vi "ColumbiaSonicareOld.vi"() -> ()   [LabVIEW 2022 SP3]
uses:
  Doppler data processing/Doppler/dopplerV6.llb/AI Waveform Scan (waveform).vi
  Doppler data processing/Doppler/dopplerV6.llb/AI Read (waveform).vi
  <vilib>/sound/lvsound.llb/Sound Format.ctl
panel:
  in  "Case Constant\n(See Context Help)":bool=TRUE
  in  "Mode":enum32{"HIFU", "Thromb"}(tab)
  out "Exp Count":i32
  in  "Time between exposures (s)":sgl=2.2 min=0 format="%.1f"
  in  "Number of Exposures":i32=1 min=1
  in  "Therapy Duration (s)":dbl=0.1 min=0.1 max=10.0 step=0.1 format="%.1f"
  out "Time":i32=1 min=1
  out "PRF time  (ms)":sgl format="%.3f"
  in  "exp per cycle  (ms)":sgl=0.5 format="%.3f"
  in  "Total  Time On (s)":sgl=1.0 min=0.001 format="%.2f"
  out "PRF  (kHz)":sgl=1.0 min=0.001 format="%.3f"
  in  "Duty Cycle":sgl=0.5 min=0 max=1 format="%.2f"
  in  "EKG ?":bool=TRUE
  in  "Re-Zero Trig":bool
  out "waveform data":waveform(dbl)[](array[waveform])
  in  "New EKG (F1)":bool
  in  "Exit Program (F2)":bool
  out "EKG":waveform(dbl)[](graph)
  in  "Fire Therapy (ESC)":bool
  out "Therapy Delay (s)":dbl=1.0 format="%.3f"
  # "1. Select EKG mode with switch below.\n2. If in EKG mode, update EKG trace with New EKG (F1).\n3. Drag pink line to mark start time of exposure and trigger level.\n4. Set time duration of exposure (0.1 s steps).\n5. Choose number of exposures and time between exposures (2.2 s min in EKG mode)..\n6. Start exposure with Fire Therapy (ESC) (Green means on).\n7. Press Fire Therapy (ESC) again for emergency stop (Red means off).\n8. To exit program, Press Exit Program (F2) to  terminate program.\n9. Thromb tab permits exposures of a fixed PRF, duty cycle, and time duration. EKG  is\n     inactive when Thromb is selected."
  # "© 2003 Riverside Research Institute"
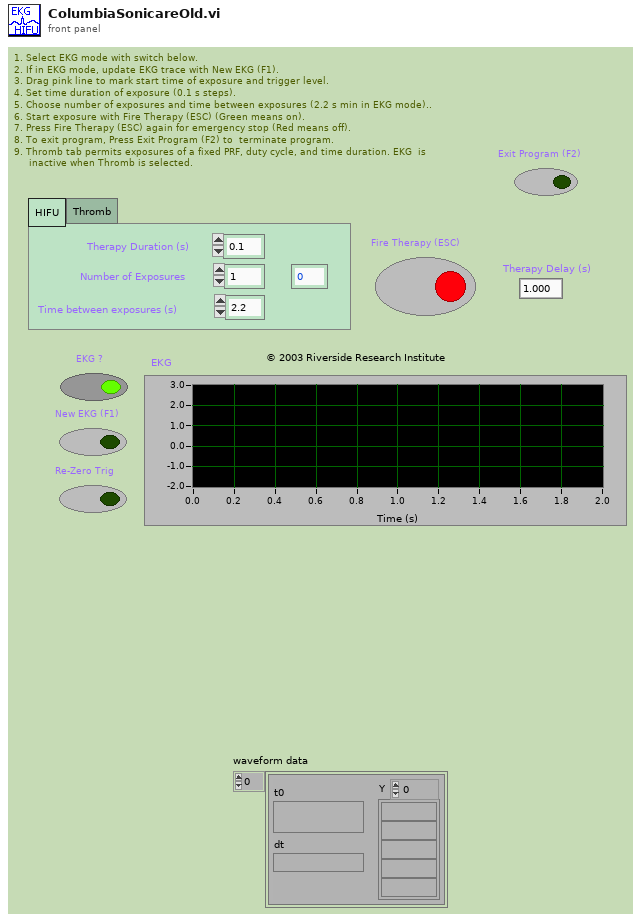
[diagram p1: front panel]
types:
  T1 = enum16{"setup mode 0", "setup mode 1", "setup mode 2", "setup mode 3", "setup mode 4", "setup mode 5", "read", "reset"}
  T2 = cluster{"coupling (no change:0)":enum16{"no change", "DC", "AC", "GND", "internal ref."}, "input config (no change:0)":u16}[]
  T3 = cluster{"high limit (0.0)":sgl, "low limit (0.0)":sgl}[]
  T4 = cluster{"trigger type (no trig:0)":enum16{"no trigger", "analog", "digital A", "digital B", "scan clock gate", "software analog "}, "pretrigger scans (0)":i32, "edge or slope \n(no change)":enum16{"no change", "rising", "falling"}, "analog chan (-) & level (0.0)":cluster{"trigger channel (empty)":string, "level (0.0)":sgl}, "scan clock source\n(no change:0)":enum16{"no change", "internal", "I/O Connector", "RTSI"}}
  T5 = typedef "Sound Format.ctl" = cluster{"sound quality":enum16{"mono", "stereo"}, "rate":enum16{"11025", "22050", "44100", "8000"}, "bits per sample":enum16{"8 bit", "16 bit"}}
  T6 = enum16{"ungated/software start", "count while high", "count while low", "start on rising edge", "start on falling edge"}
  T7 = enum16{"no trigger", "analog", "digital A", "digital A & B", "scan clock gate"}
  T8 = cluster{"trigger channel (empty)":string, "Cursor.Cursor Y":dbl}
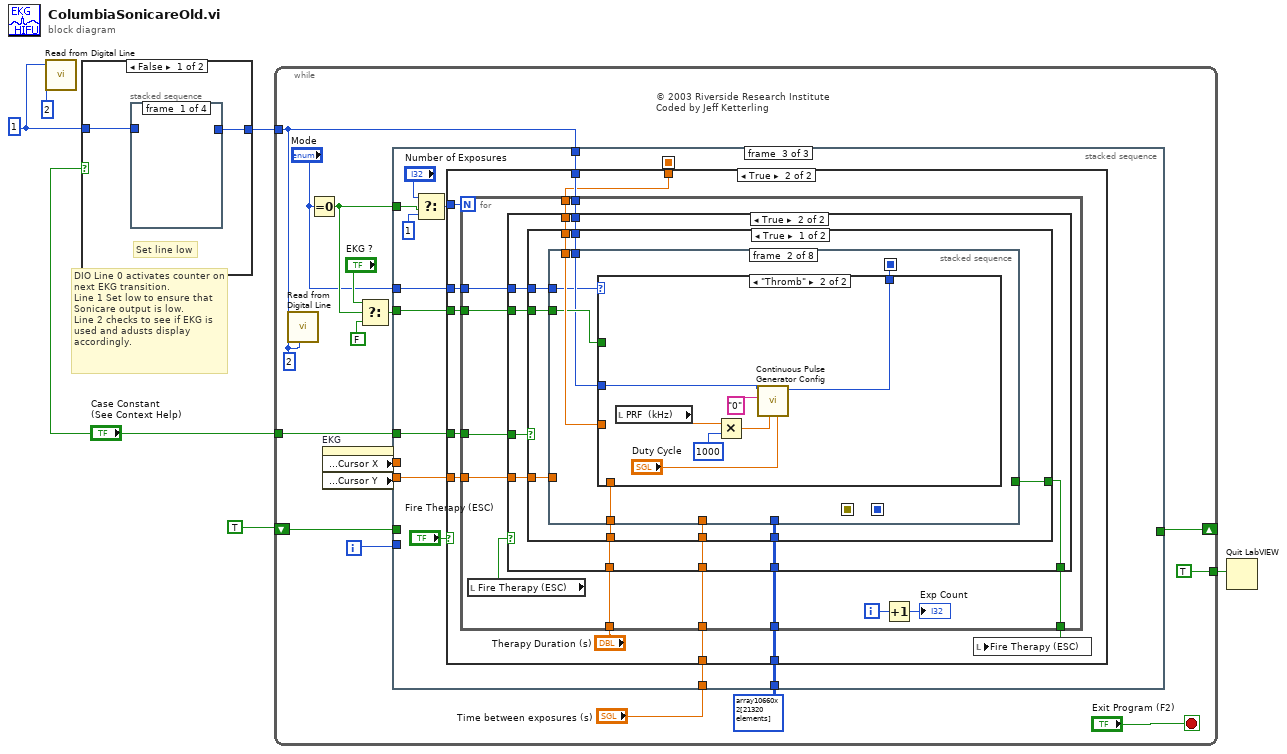
[diagram p0: block diagram]
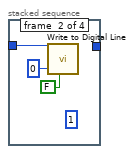
[diagram p2: hidden frame]
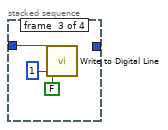
[diagram p3: hidden frame]
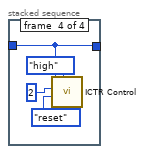
[diagram p4: hidden frame]
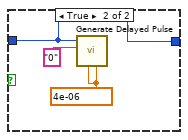
[diagram p5: hidden frame]
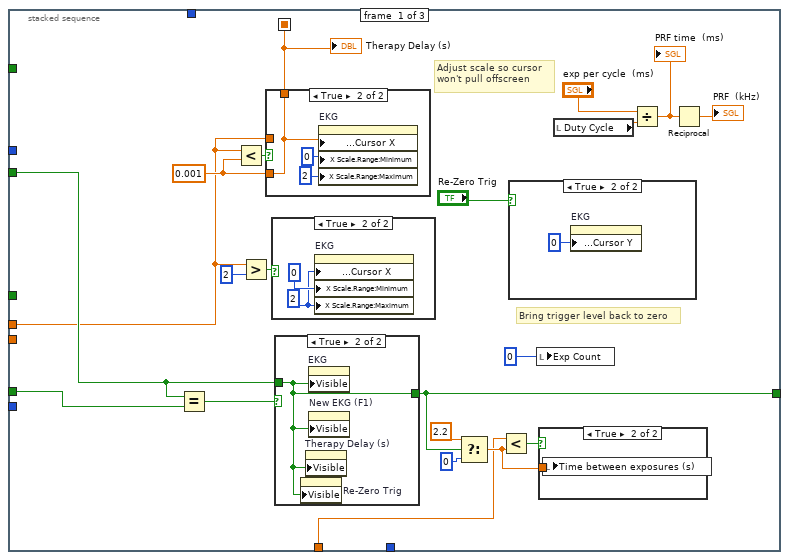
[diagram p6: hidden frame]
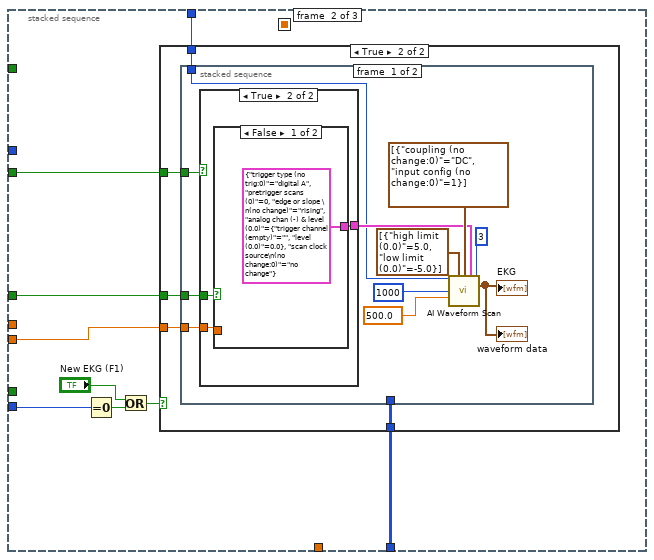
[diagram p12: hidden frame]
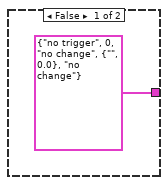
[diagram p14: hidden frame]
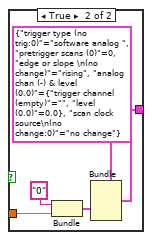
[diagram p15: hidden frame]
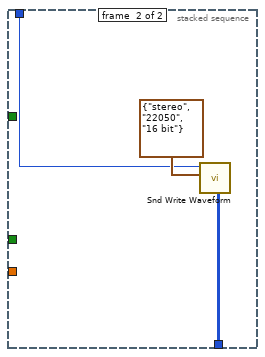
[diagram p16: hidden frame]
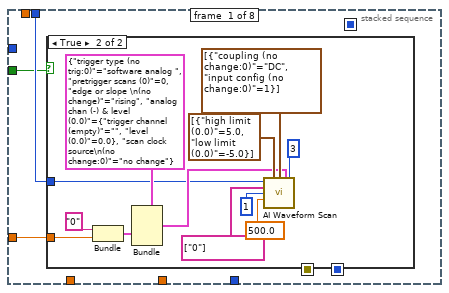
[diagram p19: hidden frame]
diagram:
  w1 = 1
  # "DIO Line 0 activates counter on next EKG transition.\nLine 1 Set low to ensure that Sonicare output is low.\nLine 2 checks to see if EKG is used and adusts display accordingly."
  n1 = call <vilib>:"Read from Digital Line.vi"("device"=w1, "line"=2) -> ()  [unwired: 5 in, 1 out]
  n2 = case shown="False" "Case Constant\n(See Context Help)" {
    tunnel: [w8 w21] -> w5
    tunnel: w1 -> [w7 w21]
    frame False {
      # "Set line low"
      n3 = stacked-sequence {
        tunnel: [_ _ _ w15] -> w8
        tunnel: w7 -> [_ w9 w13 w15]
        frame #0 {
        }
        frame #1 {
          (unwired) 1
          n4 = call <vilib>:"Write to Digital Line.vi"("device"=w9, "line"=0, "line state"=FALSE) -> ()  [unwired: 6 in]
        }
        frame #2 {
          n5 = call <vilib>:"Write to Digital Line.vi"("device"=w13, "line"=1, "line state"=FALSE) -> ()  [unwired: 6 in]
        }
        frame #3 {
          n6 = call <vilib>:"ICTR Control.vi"("output state"=enum16{"low", "high"}."high", "control code"=T1."reset", "counter"=i16 2, "device"=w15) -> ()  [unwired: 6 in, 2 out]
        }
      }
    }
    frame True {
      w19 = 4e-06
      n7 = call <vilib>:"Generate Delayed Pulse.vi"("pulse width (s or cycles)"=w19, "pulse delay (s or cycles)"=w19, "counter"="0", "device"=w21) -> ()  [unwired: 5 in, 3 out]
    }
  }
  n8 = while {
    tunnel: w5 -> [w34]
    shift-right: [w35] -> _
    shift-left: TRUE -> [w36]
    tunnel: [TRUE] -> w4
    tunnel: "Case Constant\n(See Context Help)" -> [w31]
    i -> [w37]
    stop <- "Exit Program (F2)" stop-if-true
    w32 = 2
    # "© 2003 Riverside Research Institute\nCoded by Jeff Ketterling"
    n9 = call <vilib>:"Read from Digital Line.vi"("device"=w34, "line"=w32, "iteration (0:initialize)"=w32) -> ()  [unwired: 4 in, 1 out]
    n10 = Equal To 0?(x="Mode") -> (x = 0?=w23:bool)
    n11 = property on="EKG" class="WFGraph (strict)"() -> ("Cursor.Cursor Position:Cursor X"=w29:dbl, "Cursor.Cursor Position:Cursor Y"=w30:dbl)  [unwired: 2 in, 2 out]
    n12 = Select(t="EKG ?", s=w23, f=FALSE) -> (s? t:f=w25:bool)
    n13 = stacked-sequence {
      seq-local: [w58 _ _] -> [_ _ w118]
      tunnel: w34 -> [_ w78 w120]
      tunnel: w37 -> [_ w77 _]
      tunnel: w25 -> [w54 w73 w119]
      tunnel: w36 -> [w53 _ _]
      tunnel: [w45 _ _] -> w35
      tunnel: w31 -> [_ w72 w117]
      tunnel: w30 -> [_ w71 w116]
      tunnel: w29 -> [w51 _ _]
      tunnel: i16[][] array10660x2[21320 elements] ("stereo 16-bit") -> [_ w70 w115]
      tunnel: "Time between exposures (s)" -> [w44 _ w114]
      tunnel: w23 -> [_ _ w111]
      tunnel: "Mode" -> [_ _ w108]
      frame #0 {
        w57 = 0.001
        # "Bring trigger level back to zero"
        # "Adjust scale so cursor won't pull offscreen"
        n14 = Equal?(x=w54, y=w53) -> (x = y?=w52:bool)
        n15 = Less?(x=w51, y=w57) -> (x < y?=w59:bool)
        n16 = Greater?(x=w51, y=2) -> (0:w55:bool)
        n17 = case shown="True" w59 {
          tunnel: w51 -> [w66 _]
          tunnel: [w66 w69] -> w58
          tunnel: w57 -> [_ w69]
          frame False {
          }
          frame True {
            n18 = property on="EKG" class="WFGraph (strict)"("Cursor.Cursor Position:Cursor X"=w69, "X Scale.Range:Minimum"=0, "X Scale.Range:Maximum"=2) -> ()  [unwired: 2 in, 2 out]
          }
        }
        "Therapy Delay (s)" <- w58
        n19 = case shown="True" w55 {
          frame False {
          }
          frame True {
            w64 = 2
            n20 = property on="EKG" class="WFGraph (strict)"("Cursor.Cursor Position:Cursor X"=w64, "X Scale.Range:Minimum"=0, "X Scale.Range:Maximum"=w64) -> ()  [unwired: 2 in, 2 out]
          }
        }
        n21 = case shown="True" w52 {
          tunnel: w54 -> [w62 w63]
          tunnel: [w62 w63] -> w45
          frame False {
          }
          frame True {
            n22 = property on="Re-Zero Trig" class="Bool"("Visible"=w63) -> ()  [unwired: 2 in, 2 out]
            n23 = property on="Therapy Delay (s)" class="DigNum (strict)"("Visible"=w63) -> ()  [unwired: 2 in, 2 out]
            n24 = property on="EKG" class="WFGraph (strict)"("Visible"=w63) -> ()  [unwired: 2 in, 2 out]
            n25 = property on="New EKG (F1)" class="Bool"("Visible"=w63) -> ()  [unwired: 2 in, 2 out]
          }
        }
        n26 = Select(t=2.2, s=w45, f=0) -> (s? t:f=w46:dbl)
        n27 = Less?(x=w44, y=w46) -> (x < y?=w47:bool)
        n28 = case shown="True" "Re-Zero Trig" {
          frame False {
          }
          frame True {
            n29 = property on="EKG" class="WFGraph (strict)"("Cursor.Cursor Position:Cursor Y"=0) -> ()  [unwired: 2 in, 2 out]
          }
        }
        n30 = local write "Exp Count"(0) -> ()
        n31 = case shown="True" w47 {
          tunnel: w46 -> [_ w60]
          frame False {
          }
          frame True {
            n32 = local write "Time between exposures (s)"(w60) -> ()
          }
        }
        n33 = local read "Duty Cycle"() -> (w42:sgl)
        n34 = Divide(x="exp per cycle  (ms)", y=w42) -> (x/y=w40:sgl)
        "PRF time  (ms)" <- w40
        n35 = Reciprocal(x=w40) -> (1/x=→"PRF  (kHz)":sgl)
      }
      frame #1 {
        n36 = Equal To 0?(x=w77) -> (x = 0?=w76:bool)
        n37 = Or(x="New EKG (F1)", y=w76) -> (x .or. y?=w74:bool)
        n38 = case shown="True" w74 {
          tunnel: w78 -> [_ w82]
          tunnel: w73 -> [_ w83]
          tunnel: w72 -> [_ w81]
          tunnel: w71 -> [_ w80]
          tunnel: w70 -> [_ w79]
          frame False {
          }
          frame True {
            n39 = stacked-sequence {
              tunnel: w83 -> [w87 _]
              tunnel: w82 -> [w86 w105]
              tunnel: w81 -> [w85 _]
              tunnel: w80 -> [w84 _]
              tunnel: w79 -> [_ w106]
              frame #0 {
                n40 = case shown="True" w87 {
                  tunnel: [T4 {"trigger type (no trig:0)"=enum."no trigger", "pretrigger scans (0)"=0, "edge or slope \n(no change)"=enum."no change", "analog chan (-) & level (0.0)"={"trigger channel (empty)"="", "level (0.0)"=0.0}, "scan clock source\n(no change:0)"=enum."no change"} ("trigger and clock (no trig, int clk)") w98] -> w89
                  tunnel: w85 -> [_ w97]
                  tunnel: w84 -> [_ w96]
                  frame False {
                  }
                  frame True {
                    n41 = case shown="False" w97 {
                      tunnel: [T4 {"trigger type (no trig:0)"=enum."digital A", "pretrigger scans (0)"=0, "edge or slope \n(no change)"=enum."rising", "analog chan (-) & level (0.0)"={"trigger channel (empty)"="", "level (0.0)"=0.0}, "scan clock source\n(no change:0)"=enum."no change"} ("trigger and clock (no trig, int clk)") w100] -> w98
                      tunnel: w96 -> [_ w102]
                      frame False {
                      }
                      frame True {
                        n42 = Bundle("trigger channel (empty)"="0", "Cursor.Cursor Y"=w102) -> (w103:T8)  [unwired: 1 in]
                        n43 = Bundle(cluster=T4 {"trigger type (no trig:0)"=enum."software analog ", "pretrigger scans (0)"=0, "edge or slope \n(no change)"=enum."rising", "analog chan (-) & level (0.0)"={"trigger channel (empty)"="", "level (0.0)"=0.0}, "scan clock source\n(no change:0)"=enum."no change"} ("trigger and clock (no trig, int clk)"), "analog chan (-) & level (0.0)"=w103) -> (w100:T4)  [unwired: 4 in]
                      }
                    }
                  }
                }
                n44 = call-poly "AI Waveform Scan.vi"("device (1)"=w86, "input limits (no change)"=T3 [{"high limit (0.0)"=5.0, "low limit (0.0)"=-5.0}], "coupling & input config (no change:0)"=T2 [{"coupling (no change:0)"=enum."DC", "input config (no change:0)"=1}], "trigger and clock (no trig, int clk)"=w89, "time limit in sec \n(computed:-1)"=3, "number of scans\n(1000)"=1000, "scan rate (1000 scans/sec)"=sgl 500.0) -> ("waveform data"=→"EKG" →"waveform data":waveform(dbl)[])  [unwired: 7 in, 1 out]
              }
              frame #1 {
                n45 = call <vilib>:"Snd Write Waveform.vi"("stereo 16-bit"=w106, "sound format"=T5 {"sound quality"=enum."stereo", "rate"=enum."22050", "bits per sample"=enum."16 bit"}, "device (0)"=w105) -> ()  [unwired: 8 in, 1 out]
              }
            }
          }
        }
      }
      frame #2 {
        n46 = Select(t="Number of Exposures", s=w111, f=1) -> (s? t:f=w109:i32)
        n47 = case shown="True" "Fire Therapy (ESC)" {
          tunnel: w120 -> [_ w131]
          tunnel: w119 -> [_ w130]
          tunnel: w118 -> [_ w129]
          tunnel: w109 -> [_ w128]
          tunnel: w117 -> [_ w127]
          tunnel: w116 -> [_ w126]
          tunnel: w115 -> [_ w124]
          tunnel: w114 -> [_ w123]
          tunnel: w108 -> [_ w121]
          frame False {
          }
          frame True {
            n48 = for {
              N: w128 -> [_]
              tunnel: w131 -> [w144]
              tunnel: w129 -> [w143]
              tunnel: w130 -> [w142]
              tunnel: w127 -> [w141]
              tunnel: w126 -> [w140]
              tunnel: [w139] -> w125
              tunnel: w124 -> [w138]
              tunnel: w123 -> [w136]
              tunnel: "Therapy Duration (s)" -> [w135]
              tunnel: w121 -> [w132]
              i -> [w137]
              n49 = local read "Fire Therapy (ESC)"() -> (w133:bool)
              n50 = case shown="True" w133 {
                selector: w133 -> [w145 _]
                tunnel: w144 -> [_ w155]
                tunnel: w143 -> [_ w154]
                tunnel: w142 -> [_ w153]
                tunnel: w141 -> [_ w152]
                tunnel: w140 -> [_ w151]
                tunnel: [w145 w150] -> w139
                tunnel: w138 -> [_ w149]
                tunnel: w136 -> [_ w148]
                tunnel: w135 -> [_ w147]
                tunnel: w132 -> [_ w146]
                frame False {
                }
                frame True {
                  n51 = case shown="True" w152 {
                    tunnel: w155 -> [w164 w267]
                    tunnel: w154 -> [w162 w269]
                    tunnel: [w163 w265] -> w150
                    tunnel: w147 -> [w161 w268]
                    tunnel: w153 -> [w160 w266]
                    tunnel: w151 -> [w159 _]
                    tunnel: w149 -> [w158 _]
                    tunnel: w148 -> [w157 w264]
                    tunnel: w146 -> [w156 _]
                    frame True {
                      n52 = stacked-sequence {
                        seq-local: [_ w182 _ _ _ _ _ _] -> [_ _ _ w218 w224 _ _ _]
                        seq-local: [_ _ w203 _ _ _ _ _] -> [_ _ _ _ _ w246 _ _]
                        seq-local: [_ _ w202 _ _ _ _ _] -> [_ _ _ _ _ w245 _ _]
                        tunnel: w164 -> [w167 w181 w204 _ _ _ w253 _]
                        tunnel: [_ _ _ _ w227 _ _ _] -> w163
                        tunnel: w162 -> [_ w185 _ _ w226 _ _ _]
                        tunnel: w161 -> [_ w184 _ _ w225 _ _ _]
                        tunnel: w160 -> [w166 w183 w201 _ _ w244 _ w258]
                        tunnel: w159 -> [w165 _ _ _ _ _ _ _]
                        tunnel: w158 -> [_ _ _ _ _ _ w254 _]
                        tunnel: w157 -> [_ _ _ _ _ _ _ w256]
                        tunnel: w156 -> [_ w180 _ _ w221 _ _ _]
                        frame #0 {
                          n53 = case shown="True" w166 {
                            tunnel: w167 -> [_ w169]
                            tunnel: w165 -> [_ w170]
                            frame False {
                            }
                            frame True {
                              n54 = Bundle("trigger channel (empty)"="0", "Cursor.Cursor Y"=w170) -> (w171:T8)  [unwired: 1 in]
                              n55 = Bundle(cluster=T4 {"trigger type (no trig:0)"=enum."software analog ", "pretrigger scans (0)"=0, "edge or slope \n(no change)"=enum."rising", "analog chan (-) & level (0.0)"={"trigger channel (empty)"="", "level (0.0)"=0.0}, "scan clock source\n(no change:0)"=enum."no change"} ("trigger and clock (no trig, int clk)"), "analog chan (-) & level (0.0)"=w171) -> (w173:T4)  [unwired: 4 in]
                              n56 = call-poly "AI Waveform Scan.vi"("device (1)"=w169, "input limits (no change)"=T3 [{"high limit (0.0)"=5.0, "low limit (0.0)"=-5.0}], "coupling & input config (no change:0)"=T2 [{"coupling (no change:0)"=enum."DC", "input config (no change:0)"=1}], "trigger and clock (no trig, int clk)"=w173, "time limit in sec \n(computed:-1)"=3, "channels (0)"=tag[] ["0"], "number of scans\n(1000)"=1, "scan rate (1000 scans/sec)"=sgl 500.0) -> ()  [unwired: 6 in, 2 out]
                            }
                          }
                        }
                        frame #1 {
                          n57 = case shown="\"Thromb\"" w180 {
                            tunnel: w185 -> [w192 _]
                            tunnel: w184 -> [w191 _]
                            tunnel: w183 -> [w189 _]
                            tunnel: [w188 w198] -> w182
                            tunnel: w181 -> [w187 w199]
                            frame "HIFU", Default {
                              w186 = T6."ungated/software start" ("gate mode (ungated:0)")
                              # "For use with normal NI DAQ E series sardware"
                              n58 = Select(t=T6."start on rising edge" ("gate mode (ungated:0)"), s=w189, f=w186) -> ()  [unwired: 1 out]
                              n59 = call <vilib>:"Generate Delayed Pulse.vi"("pulse width (s or cycles)"=w191, "pulse delay (s or cycles)"=w192, "gate mode (ungated:0)"=w186, "counter"="0", "device"=w187) -> ("[taskID]"=w188:u32)  [unwired: 4 in, 2 out]
                            }
                            frame "Thromb" {
                              n60 = local read "PRF  (kHz)"() -> (w194:sgl)
                              n61 = Multiply(x=w194, y=1000) -> (x*y=w196:sgl)
                              n62 = call <vilib>:"Continuous Pulse Generator Config.vi"("duty cycle (0.5)"="Duty Cycle", "frequency (Hz)"=w196, "counter"="0", "device"=w199) -> ("taskID"=w198:u32)  [unwired: 4 in, 3 out]
                            }
                          }
                        }
                        frame #2 {
                          n63 = case shown="False" w201 {
                            tunnel: w204 -> [_ w210]
                            tunnel: [u32 0 ("taskID out") w209] -> w203
                            tunnel: [errorcluster {"status"=FALSE, "code"=0, "source"=""} ("error out") w208] -> w202
                            frame False {
                            }
                            frame True {
                              n64 = call "AI Config.vi"("device (1)"=w210, "input limits (no change)"=T3 [{"high limit (0.0)"=5.0, "low limit (0.0)"=-5.0}], "channels (0)"=tag[] ["0,1"], "buffer size (1000 scans)"=1000, "[group] (0)"=1) -> ("taskID"=w212:u32, "error out"=w217:errorcluster)  [unwired: 8 in, 1 out]
                              n65 = call "AI Start.vi"("taskID in"=w212, "trigger type (no trig:0)"=T7."no trigger", "scan rate (1000 scans/sec)"=sgl 500.0, "error in (no error)"=w217) -> ("taskID out"=w209:u32, "error out"=w208:errorcluster)  [unwired: 8 in, 2 out]
                            }
                          }
                        }
                        frame #3 {
                          n66 = call <vilib>:"Counter Start.vi"("taskID"=w218) -> ()  [unwired: 9 in, 2 out]
                        }
                        frame #4 {
                          n67 = Not Equal To 0?(x=w221) -> (x != 0?=w223:bool)
                          n68 = Add(x=w226, y=w225) -> (x+y=w220:dbl)
                          n69 = Select(t="Total  Time On (s)", s=w223, f=w220) -> (s? t:f=w219:dbl)
                          n70 = Multiply(x=w219, y=1000) -> (x*y=w228:dbl)
                          n71 = Tick Count (ms)() -> (millisecond timer value=w230:u32)
                          n72 = while {
                            tunnel: w224 -> [w242]
                            tunnel: w230 -> [w240]
                            tunnel: w228 -> [w239]
                            tunnel: [FALSE] -> w227
                            stop <- w234 stop-if-true
                            # "Stop if aborted or time limit up"
                            n73 = local read "Fire Therapy (ESC)"() -> (w236:bool)
                            n74 = Tick Count (ms)() -> (millisecond timer value=w241:u32)
                            n75 = Subtract(x=w241, y=w240) -> (x-y=w233:u32)
                            n76 = Greater?(x=w233, y=w239) -> (0:w238:bool)
                            n77 = Not(x=w236) -> (.not. x?=w235:bool)
                            n78 = Divide(x=w233, y=1000) -> (x/y=→"Time":dbl)
                            n79 = Or(x=w235, y=w238) -> (x .or. y?=w234:bool)
                            n80 = case shown="True" w234 {
                              tunnel: w242 -> [_ w243]
                              frame False {
                              }
                              frame True {
                                n81 = call <vilib>:"Counter Stop.vi"("taskID"=w243) -> ()  [unwired: 5 in, 2 out]
                              }
                            }
                          }
                        }
                        frame #5 {
                          n82 = case shown="True" w244 {
                            tunnel: w246 -> [_ w248]
                            tunnel: w245 -> [_ w247]
                            frame False {
                            }
                            frame True {
                              n83 = call-poly "AI Read.vi"("taskID in"=w248, "number of scans to read (-1:all)"=1000, "error in (no error)"=w247) -> ("taskID out"=w251:u32, "waveform data"=w249:waveform(dbl)[], "error out"=w250:errorcluster)  [unwired: 7 in, 3 out]
                              n84 = local write "EKG"(w249) -> ()
                              n85 = call "AI Clear.vi"("error in (no error)"=w250, "taskID in"=w251) -> ()  [unwired: 4 in, 2 out]
                            }
                          }
                        }
                        frame #6 {
                          n86 = call <vilib>:"Snd Write Waveform.vi"("stereo 16-bit"=w254, "sound format"=T5 {"sound quality"=enum."stereo", "rate"=enum."22050", "bits per sample"=enum."16 bit"}, "device (0)"=w253) -> ()  [unwired: 8 in, 1 out]
                        }
                        frame #7 {
                          n87 = Select(t=2.2, s=w258, f=0) -> (s? t:f=w259:dbl)
                          n88 = Subtract(x=w256, y=w259) -> (x-y=w262:dbl)
                          n89 = Multiply(x=w262, y=1000) -> (x*y=w261:dbl)
                          n90 = Wait (ms)(milliseconds to wait=w261) -> ()  [unwired: 1 out]
                        }
                      }
                    }
                    frame False {
                      n91 = stacked-sequence {
                        seq-local: [w275 _ _ _ _ _ _ _] -> [_ _ _ _ _ _ w330 _]
                        seq-local: [w274 _ _ _ _ _ _ _] -> [_ _ _ _ _ _ w328 _]
                        tunnel: w269 -> [_ w285 _ w304 _ _ _ _]
                        tunnel: w268 -> [_ w284 _ w294 _ _ _ _]
                        tunnel: w267 -> [w278 w283 w289 w299 w320 _ _ _]
                        tunnel: w266 -> [_ w282 _ w292 _ _ _ _]
                        tunnel: [_ _ _ w300 _ _ _ _] -> w265
                        tunnel: [_ w281 _ _ _ _ _ _] -> _
                        tunnel: w264 -> [_ _ _ _ _ _ _ w331]
                        frame #0 {
                          n92 = call "AI Config.vi"("device (1)"=w278, "input limits (no change)"=T3 [{"high limit (0.0)"=5.0, "low limit (0.0)"=-5.0}], "channels (0)"=tag[] ["2"], "buffer size (1000 scans)"=1000, "[group] (0)"=1) -> ("taskID"=w271:u32, "error out"=w280:errorcluster)  [unwired: 8 in, 1 out]
                          n93 = call "AI Start.vi"("taskID in"=w271, "trigger type (no trig:0)"=T7."digital A", "scan rate (1000 scans/sec)"=sgl 500.0, "error in (no error)"=w280) -> ("taskID out"=w275:u32, "error out"=w274:errorcluster)  [unwired: 8 in, 2 out]
                        }
                        frame #1 {
                          # "Make Sure timers are set up before next frame"
                          # "For Use with DAQ-1200 timer chip"
                          n94 = call "PulseGenDigStart8253.vi"("device"=w283, "Gate Start?"=w282, "pulse delay (s)"=w285, "pulse width (s)"=w284) -> ("actual width (s)"=w281:dbl)  [unwired: 10 in, 1 out]
                        }
                        frame #2 {
                          # "Set line high. Flip flop will then gate timer on next sync pulse"
                          n95 = call <vilib>:"Write to Digital Line.vi"("device"=w289, "line"=0, "line state"=TRUE, "iteration (0:initialize)"=1) -> ()  [unwired: 5 in]
                        }
                        frame #3 {
                          n96 = Select(t=1, s=w292, f=0.1) -> (s? t:f=w293:dbl)
                          n97 = Compound Arithmetic op=ADD(w293, w304, w294) -> (w307:dbl)
                          n98 = Multiply(x=w307, y=1000) -> (x*y=w305:dbl)
                          n99 = Tick Count (ms)() -> (millisecond timer value=w308:u32)
                          n100 = while {
                            tunnel: w308 -> [w317]
                            tunnel: w305 -> [w315]
                            tunnel: [FALSE] -> w300
                            tunnel: [w309] -> w295
                            tunnel: w299 -> [w309]
                            stop <- w313 stop-if-true
                            n101 = local read "Fire Therapy (ESC)"() -> (w311:bool)
                            n102 = Tick Count (ms)() -> (millisecond timer value=w318:u32)
                            n103 = Subtract(x=w318, y=w317) -> (x-y=w316:u32)
                            n104 = Not(x=w311) -> (.not. x?=w310:bool)
                            n105 = Greater?(x=w316, y=w315) -> (0:w314:bool)
                            n106 = Or(x=w310, y=w314) -> (x .or. y?=w313:bool)
                          }
                          n107 = call <vilib>:"ICTR Control.vi"("output state"=enum16{"low", "high"}."high", "control code"=T1."reset", "counter"=i16 2, "device"=w295) -> ()  [unwired: 6 in, 2 out]
                          n108 = call <vilib>:"ICTR Control.vi"("output state"=enum16{"low", "high"}."high", "control code"=T1."reset", "counter"=i16 1, "device"=w295) -> ()  [unwired: 6 in, 2 out]
                        }
                        frame #4 {
                          # "Set line low to turn of gate signal to counter"
                          n109 = call <vilib>:"Write to Digital Line.vi"("device"=w320, "line"=0, "line state"=FALSE, "iteration (0:initialize)"=1) -> ()  [unwired: 5 in]
                        }
                        frame #5 {
                          n110 = call <vilib>:"Beep.vi"() -> ()  [unwired: 12 in]
                        }
                        frame #6 {
                          n111 = local read "waveform data"() -> (w323:waveform(dbl)[])
                          n112 = call-poly "AI Read.vi"("taskID in"=w330, "number of scans to read (-1:all)"=1000, "error in (no error)"=w328) -> ("taskID out"=w327:u32, "waveform data"=w325:waveform(dbl)[], "error out"=w326:errorcluster)  [unwired: 7 in, 3 out]
                          n113 = Build Array (concatenate)(w323, w325) -> (w324:waveform(dbl)[])
                          n114 = call "AI Clear.vi"("error in (no error)"=w326, "taskID in"=w327) -> ()  [unwired: 4 in, 2 out]
                          n115 = local write "EKG"(w324) -> ()
                        }
                        frame #7 {
                          n116 = Subtract(x=w331, y=2) -> (x-y=w332:sgl)
                          n117 = Multiply(x=w332, y=1000) -> (x*y=w334:sgl)
                          n118 = Wait (ms)(milliseconds to wait=w334) -> ()  [unwired: 1 out]
                        }
                      }
                    }
                  }
                }
              }
              n119 = Increment(x=w137) -> (x+1=→"Exp Count":i32)
            }
            n120 = local write "Fire Therapy (ESC)"(w125) -> ()
          }
        }
      }
    }
  }
  n121 = Quit LabVIEW(quit? (T)=w4) -> ()
